vi "updateHoloBundle.vi"(8 "NewValue":variant, 9 "input cluster":T1={"1_Radio"=enum."Radio Selection 2", "1_Trans"=100.0, "1_Phase"=0.0, "HoloCode 1"="", "1_Semi"=FALSE, "1_Active"=0, "1_ModType"="_complex", "1_Flip"="no flip", "HoloNum"=0.0, "ParamStr"="", "ParamVal"=0.0, "ParamAux"=""} {"1_Phase" scale=0.0..360.0; "1_Trans" scale=0.0..100.0}, 11 "CtlRef":refnum<vi>) -> (1 "output cluster":T1, 3 "substring":string)   [LabVIEW 2023]
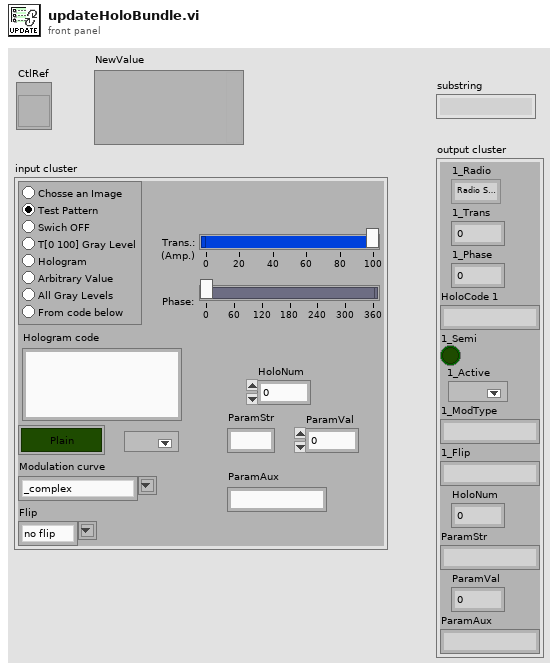
[diagram p1: front panel]
types:
  T1 = cluster{"1_Radio":enum32{"Radio Selection 1", "Radio Selection 2", "Radio Selection 3", "Radio Selection 4", "Radio Selection 5", "Radio Selection 6", "Radio Selection 7", "Radio Selection 8"}, "1_Trans":dbl, "1_Phase":dbl, "HoloCode 1":string, "1_Semi":bool, "1_Active":u16, "1_ModType":string, "1_Flip":string, "HoloNum":dbl, "ParamStr":string, "ParamVal":dbl, "ParamAux":string}
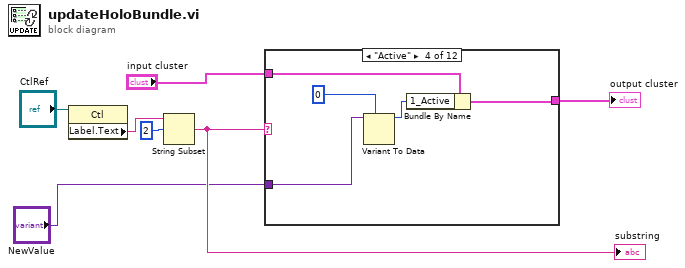
[diagram p0: block diagram]
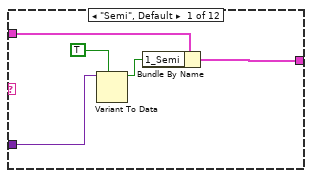
[diagram p2: hidden frame]
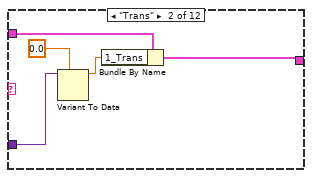
[diagram p3: hidden frame]
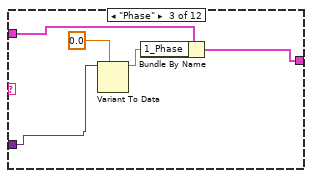
[diagram p4: hidden frame]
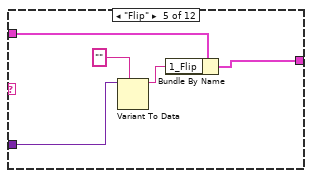
[diagram p5: hidden frame]
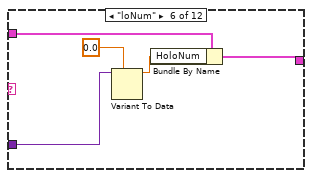
[diagram p6: hidden frame]
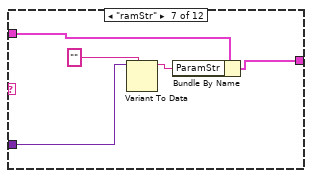
[diagram p7: hidden frame]
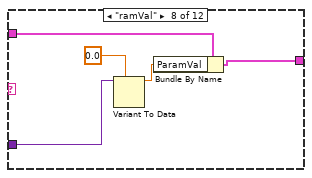
[diagram p8: hidden frame]
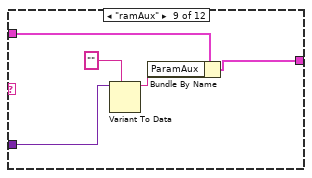
[diagram p9: hidden frame]
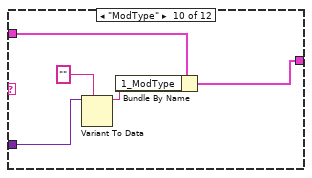
[diagram p10: hidden frame]
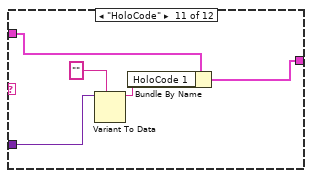
[diagram p11: hidden frame]
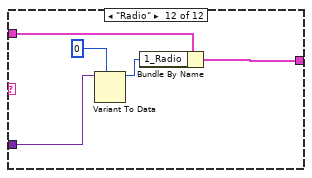
[diagram p12: hidden frame]
diagram:
  n1 = property class="Ctl"(reference="CtlRef") -> ("Label.Text"=w5:string)  [unwired: 1 in, 2 out]
  n2 = String Subset(string=w5, offset (0)=2) -> (substring=w3:string)  [unwired: 1 in]
  "substring" <- w3
  n3 = case shown="\"Active\"" w3 {
    tunnel: "input cluster" -> [w10 w14 w18 w25 w29 w34 w39 w44 w49 w55 w60 w67]
    tunnel: [w9 w15 w19 w26 w30 w35 w40 w45 w48 w54 w59 w66] -> w1
    tunnel: "NewValue" -> [w8 w13 w20 w24 w28 w33 w38 w43 w50 w53 w58 w63]
    frame "Semi", Default {
      n4 = Variant To Data(type=TRUE, Variant=w8) -> (data=w11:bool)  [unwired: 1 in, 1 out]
      n5 = Bundle By Name(cluster=w10, "1_Semi"=w11) -> (w9:T1)
    }
    frame "Trans" {
      n6 = Variant To Data(type=0.0, Variant=w13) -> (data=w16:dbl)  [unwired: 1 in, 1 out]
      n7 = Bundle By Name(cluster=w14, "1_Trans"=w16) -> (w15:T1)
    }
    frame "Phase" {
      n8 = Variant To Data(type=0.0, Variant=w20) -> (data=w21:dbl)  [unwired: 1 in, 1 out]
      n9 = Bundle By Name(cluster=w18, "1_Phase"=w21) -> (w19:T1)
    }
    frame "Active" {
      n10 = Variant To Data(type=0, Variant=w24) -> (data=w27:i32)  [unwired: 1 in, 1 out]
      n11 = Bundle By Name(cluster=w25, "1_Active"=w27) -> (w26:T1)
    }
    frame "Flip" {
      n12 = Variant To Data(type="", Variant=w28) -> (data=w31:string)  [unwired: 1 in, 1 out]
      n13 = Bundle By Name(cluster=w29, "1_Flip"=w31) -> (w30:T1)
    }
    frame "loNum" {
      n14 = Variant To Data(type=0.0, Variant=w33) -> (data=w36:dbl)  [unwired: 1 in, 1 out]
      n15 = Bundle By Name(cluster=w34, "HoloNum"=w36) -> (w35:T1)
    }
    frame "ramStr" {
      n16 = Variant To Data(type="", Variant=w38) -> (data=w41:string)  [unwired: 1 in, 1 out]
      n17 = Bundle By Name(cluster=w39, "ParamStr"=w41) -> (w40:T1)
    }
    frame "ramVal" {
      n18 = Variant To Data(type=0.0, Variant=w43) -> (data=w46:dbl)  [unwired: 1 in, 1 out]
      n19 = Bundle By Name(cluster=w44, "ParamVal"=w46) -> (w45:T1)
    }
    frame "ramAux" {
      n20 = Variant To Data(type="", Variant=w50) -> (data=w51:string)  [unwired: 1 in, 1 out]
      n21 = Bundle By Name(cluster=w49, "ParamAux"=w51) -> (w48:T1)
    }
    frame "ModType" {
      n22 = Variant To Data(type="", Variant=w53) -> (data=w56:string)  [unwired: 1 in, 1 out]
      n23 = Bundle By Name(cluster=w55, "1_ModType"=w56) -> (w54:T1)
    }
    frame "HoloCode" {
      n24 = Variant To Data(type="", Variant=w58) -> (data=w61:string)  [unwired: 1 in, 1 out]
      n25 = Bundle By Name(cluster=w60, "HoloCode 1"=w61) -> (w59:T1)
    }
    frame "Radio" {
      n26 = Variant To Data(type=u32 0, Variant=w63) -> (data=w64:u32)  [unwired: 1 in, 1 out]
      n27 = Bundle By Name(cluster=w67, "1_Radio"=w64) -> (w66:T1)
    }
  }
  "output cluster" <- w1
